vi "WPI_IMU_ADIS16460_FGV.vi"(0 "ADI IMU Interrupt DevRef":T2={"ADI IMU DevRef"={"DevStatus"={"status"=FALSE, "code"=0, "source"=""}, "Handle"=0, "SPI Bus"=enum."SPI On-Board, CS0", "Device Found"=FALSE, "Device Ready"=FALSE, "Yaw Axis"=enum."Z", "AHRS Algorithm"=enum."Complementary"}, "InterruptRef"={"DevStatus"={"status"=FALSE, "code"=0, "source"=""}, "InterruptIndex"=enum."0"}}, 1 "Operation":enum16{"set", "get"}(ring), 2 "Sensor Ready?":bool, 5 "Reset":bool, 7 "IMU Data":T1, 9 "IMU Angles":T7, 11 "IMU AHRS":cluster{"Pitch":dbl, "Roll":dbl}) -> (4 "ADI IMU Interrupt DevRef":T2={"ADI IMU DevRef"={"DevStatus"={"status"=FALSE, "code"=0, "source"=""}, "Handle"=0, "SPI Bus"=enum."SPI On-Board, CS0", "Device Found"=FALSE, "Device Ready"=FALSE, "Yaw Axis"=enum."Z", "AHRS Algorithm"=enum."Complementary"}, "InterruptRef"={"DevStatus"={"status"=FALSE, "code"=0, "source"=""}, "InterruptIndex"=enum."0"}}, 6 "Reset Out":bool, 8 "IMU Data Out":T1, 10 "IMU Angles Out":T7, 13 "Sensor Ready Out":bool, 15 "IMU AHRS OUT":cluster{"Pitch":dbl, "Roll":dbl})   [LabVIEW 2015, in "FRC ADIS16460.lvlib"]
uses:
  FRC ADIS16460.lvlib
  WPI_ADIS16460_InterruptDevRef.ctl
  WPI_ADIS16460_DevRef.ctl
  <vilib>/Rock Robotics/SystemInterfaces/spilib/spi_bus.ctl
  <vilib>/Rock Robotics/WPI/Interrupt/WPI_InterruptRef.ctl
  <vilib>/Rock Robotics/SystemInterfaces/Interrupt/FPGA_InterruptIndex.ctl
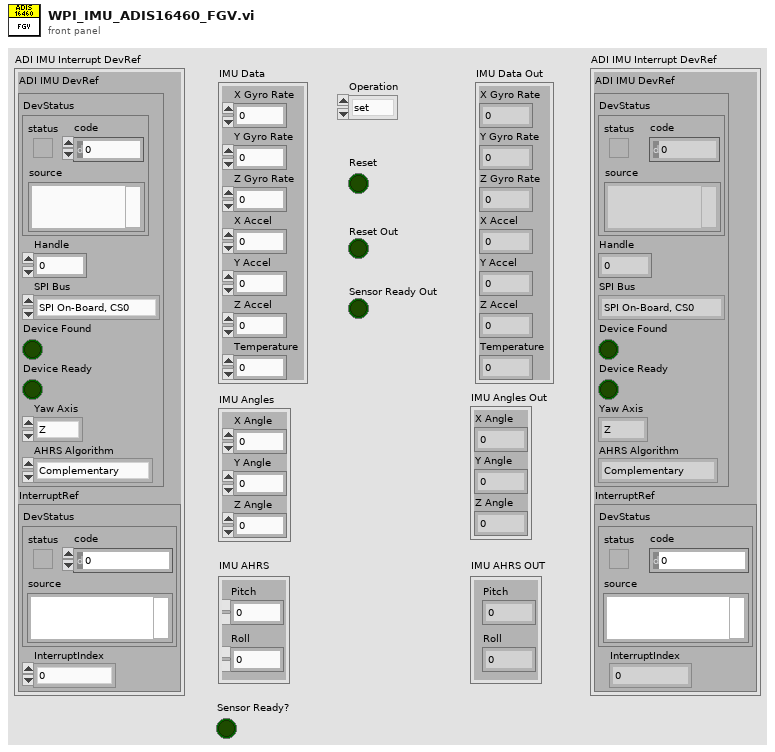
[diagram p1: front panel]
types:
  T1 = cluster{"X Gyro Rate":dbl, "Y Gyro Rate":dbl, "Z Gyro Rate":dbl, "X Accel":dbl, "Y Accel":dbl, "Z Accel":dbl, "Temperature":dbl}
  T2 = typedef "FRC ADIS16460.lvlib/WPI_ADIS16460_InterruptDevRef.ctl" = cluster{"ADI IMU DevRef":T3, "InterruptRef":T5}
  T3 = typedef "FRC ADIS16460.lvlib/WPI_ADIS16460_DevRef.ctl" = cluster{"DevStatus":errorcluster, "Handle":i32, "SPI Bus":T4, "Device Found":bool, "Device Ready":bool, "Yaw Axis":enum16{"X", "Y", "Z"}, "AHRS Algorithm":enum16{"Complementary", "Madgwick"}}
  T4 = typedef "spi_bus.ctl" = enum16{"SPI On-Board, CS0", "SPI On-Board, CS1", "SPI On-Board, CS2", "SPI On-Board, CS3", "SPI MXP", "Invalid"}
  T5 = typedef "WPI_InterruptRef.ctl" = cluster{"DevStatus":errorcluster, "InterruptIndex":T6}
  T6 = typedef "FPGA_InterruptIndex.ctl" = enum8{"0", "1", "2", "3", "4", "5", "6", "7", "Invalid"}
  T7 = cluster{"X Angle":dbl, "Y Angle":dbl, "Z Angle":dbl}
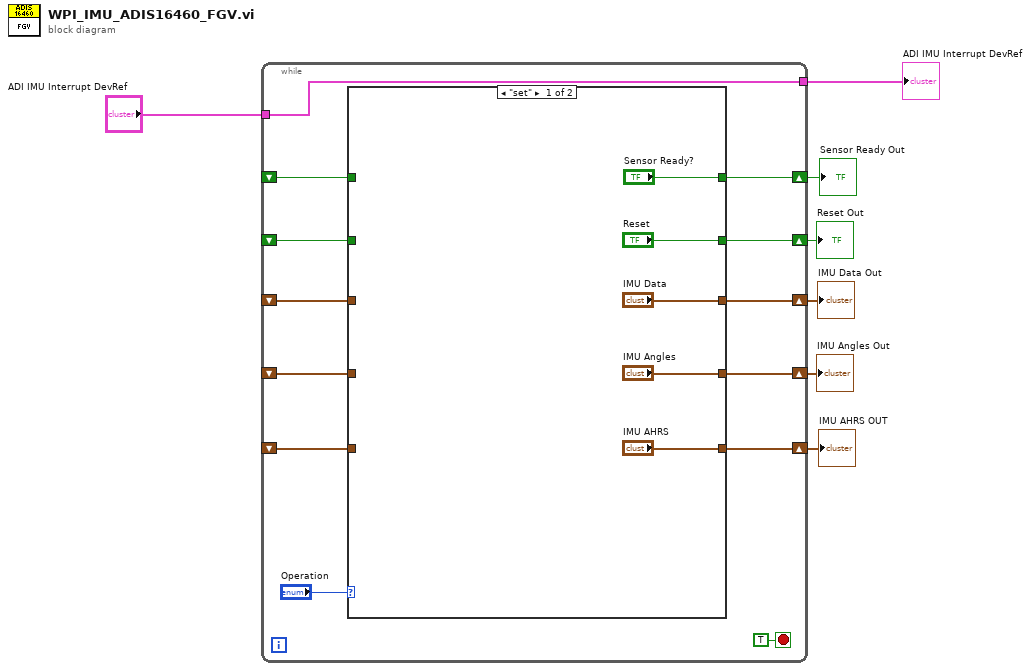
[diagram p0: block diagram]
diagram:
  n1 = while {
    shift-right: [w18] -> w7
    shift-left: _ -> [w12]
    shift-right: [w17] -> w1
    shift-left: _ -> [w13]
    tunnel: "ADI IMU Interrupt DevRef" -> [w16]
    tunnel: [w16] -> w3
    shift-right: [w15] -> w6
    shift-left: _ -> [w14]
    shift-right: [w11] -> w2
    shift-left: _ -> [w10]
    shift-right: [w9] -> w5
    shift-left: _ -> [w8]
    stop <- TRUE stop-if-true
    n2 = case shown="\"set\"" "Operation" {
      tunnel: ["Reset" w28] -> w18
      tunnel: ["IMU Data" w29] -> w17
      tunnel: ["IMU Angles" w30] -> w15
      tunnel: w14 -> [_ w30]
      tunnel: w13 -> [_ w29]
      tunnel: w12 -> [_ w28]
      tunnel: ["IMU AHRS" w27] -> w11
      tunnel: w10 -> [_ w27]
      tunnel: ["Sensor Ready?" w26] -> w9
      tunnel: w8 -> [_ w26]
      frame "set" {
      }
      frame "get", Default {
      }
    }
  }
  "Reset Out" <- w7
  "IMU Angles Out" <- w6
  "Sensor Ready Out" <- w5
  "ADI IMU Interrupt DevRef" <- w3
  "IMU AHRS OUT" <- w2
  "IMU Data Out" <- w1
